vi "ENPH354_LabTracers2.vi"() -> ()   [LabVIEW 2020]
uses:
  1e4b00a4-0517-4322-bb3b-720fe8f45536.vi
  <vilib>/MakerHub/LINX/Public/Peripherals/PWM/PWM Set Duty Cycle 1 Chan.vi
  <vilib>/MakerHub/LINX/Public/Peripherals/Digital/Digital Write 1 Chan.vi
  75366657-9a63-4780-a10d-0fe28d3ec2d1.vi
  8bd6eaf3-79a2-4ca0-8ca0-17b2d510817e.vi
  <vilib>/MakerHub/LINX/Public/Peripherals/Analog/Analog Read 1 Chan.vi
  ab133cba-5ad7-442c-8e32-8a5f556f998e.vi
  <vilib>/MakerHub/LINX/Public/Peripherals/Digital/Digital Write N Chans.vi
  <vilib>/MakerHub/LINX/Public/Peripherals/Analog/Analog Read N Chans.vi
  <vilib>/MakerHub/LINX/Private/Local IO/LinxDigitalWrite.vi
  <vilib>/MakerHub/LINX/Public/Utilities/Check Channel.vi
  <vilib>/MakerHub/LINX/Private/Local IO/LinxAnalogRead.vi
  <vilib>/MakerHub/LINX/Public/Utilities/Open Serial.vi
  <vilib>/MakerHub/LINX/Public/Peripherals/PWM/PWM Set Duty Cycle N Chans.vi
  <vilib>/MakerHub/LINX/Private/Utilties/Generate Error.vi
  <vilib>/MakerHub/LINX/LMH-LINX.lvlib
panel:
  in  "Final Motor Angle [deg]":dbl
  in  "Initial Motor Angle [deg]":dbl
  in  "Motor Step Size [deg]":dbl
  in  "Voltage Step Size [V]":dbl
  out "PCE(n) [%]":dbl
  out "R_sh [Ohm]":dbl
  out "R_s [Ohm]":dbl
  out "FF":dbl
  out "V_oc [V]":dbl
  out "I_sc [A]":dbl
  out "Index":dbl
  out "Light Index":dbl
  out "Dark Index":dbl
  out "AVG Current SC [mA]":dbl
  out "AVG Current Light [mA]":dbl
  out "AVG Current Dark [mA]":dbl
  out "Duty Cycle":dbl
  out "AVG Bias V":dbl
  in  "Save Incident Angle Data":path
  in  "Save Dark IV Data":path
  in  "Save Light IV SCPE":path
  in  "Save Light IV Data":path
  in  "Skip Light":bool
  in  "Skip L&D":bool
  in  "Skip Dark":bool
  out "Short Circuit Current vs Incident Angle":cluster{"X":dbl[], "Y":dbl[]}[](graph)
  in  "stop 2":bool
  out "LED On":bool
  out "Light IV":cluster{"X":dbl[], "Y":dbl[]}[](graph)
  out "error out":errorcluster
  in  "stop":bool
  out "Bias Voltage":dbl(graph)
  out "Dark IV":cluster{"X":dbl[], "Y":dbl[]}[](graph)
  # "Press the \"Skip\" before executing"
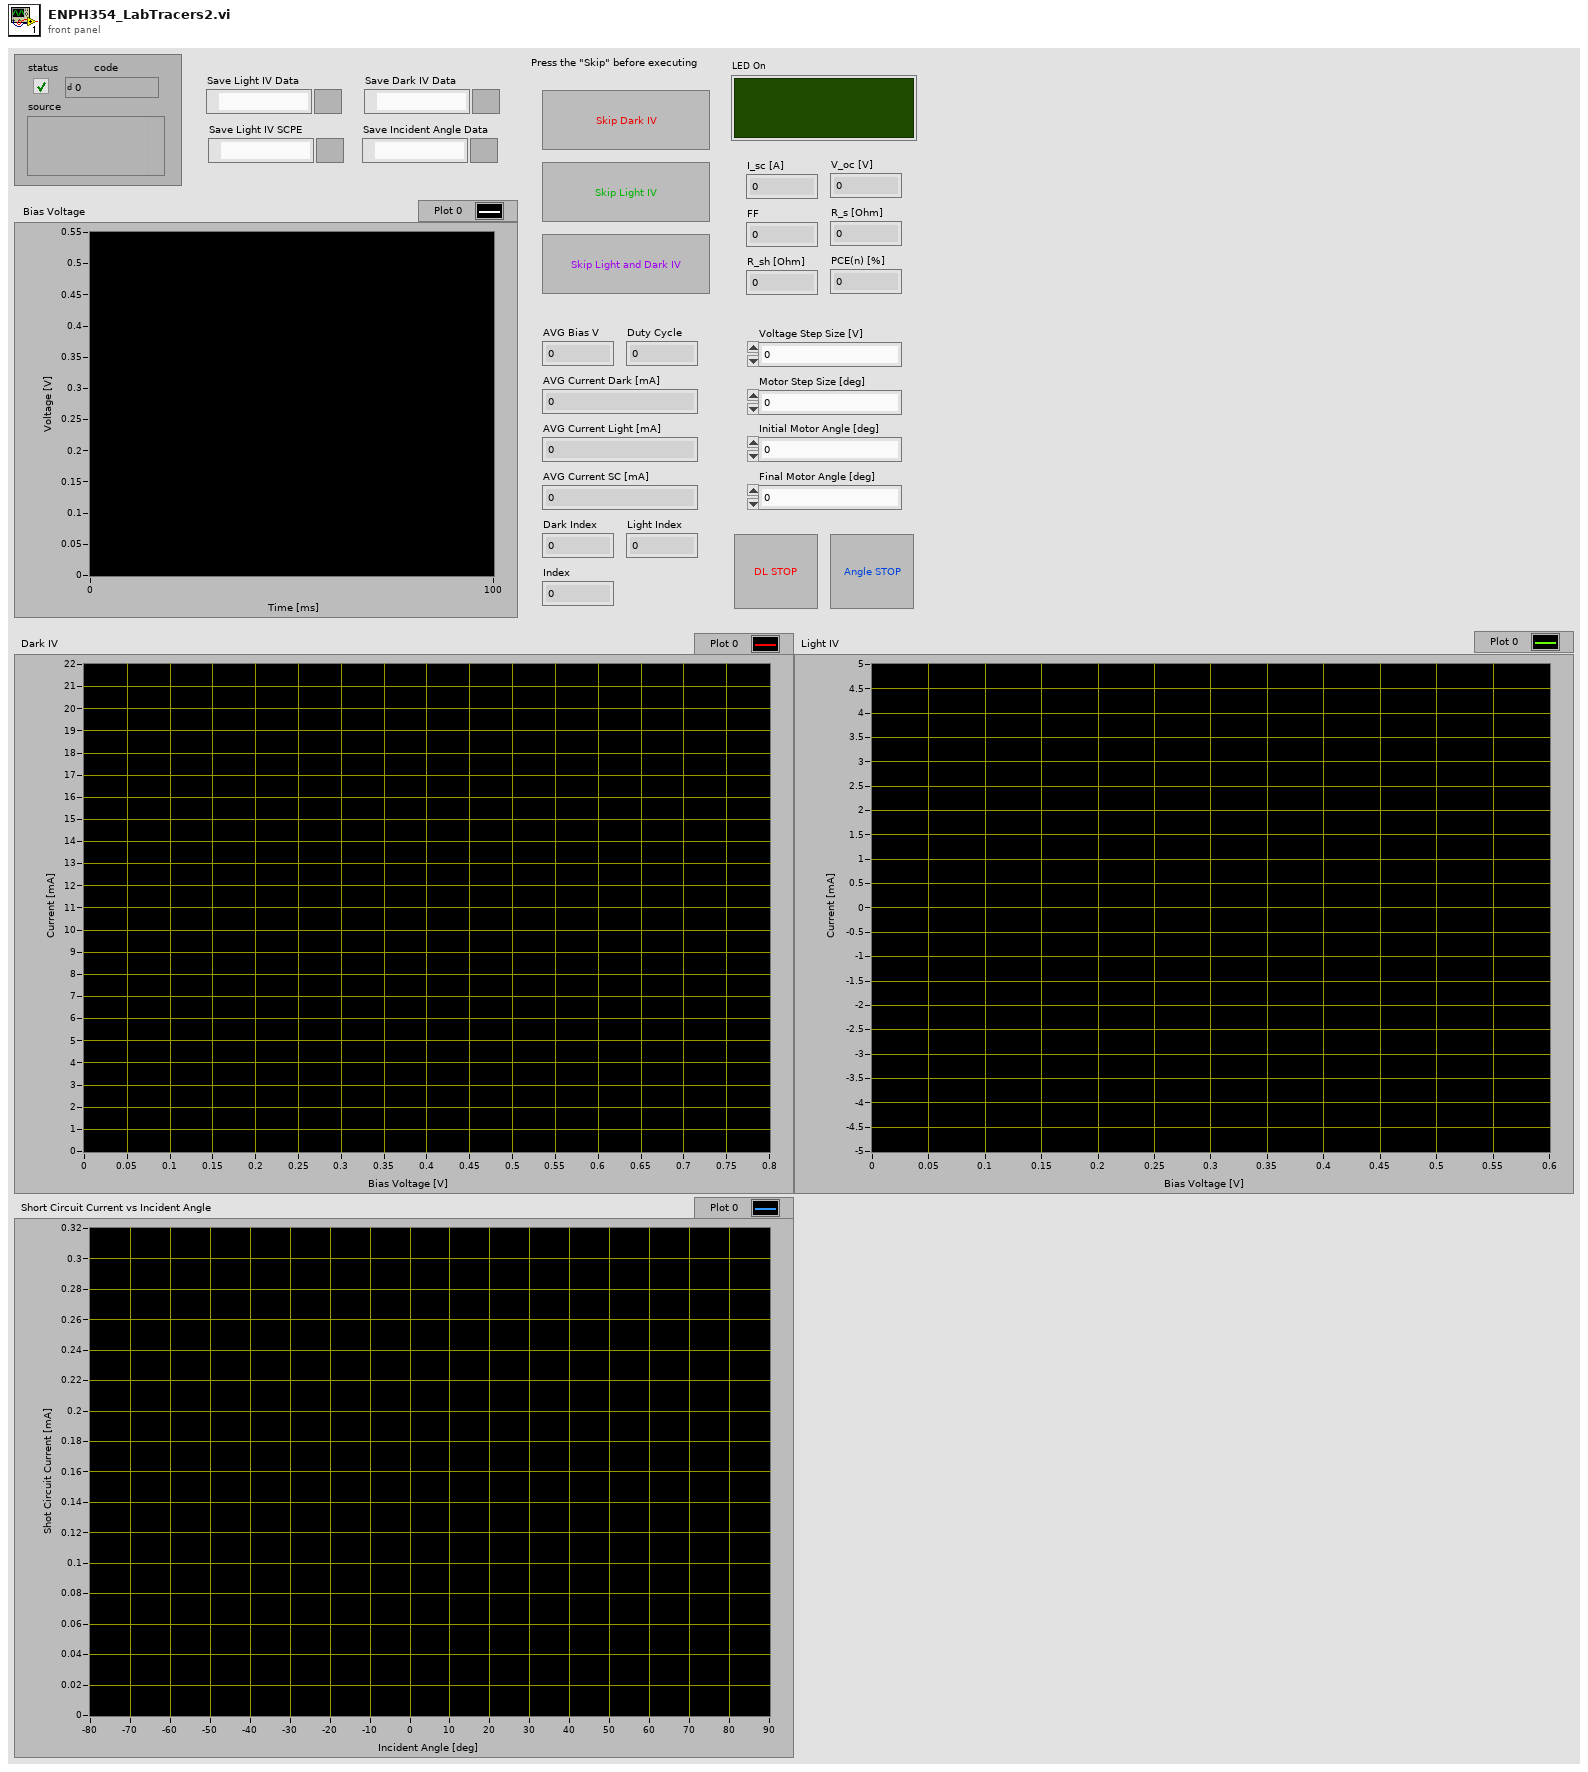
[diagram p1: front panel]
types:
  T1 = typedef "LMH-LINX.lvlib/LINX Ref.ctl" = cluster{"IO":T2, "Interface":T3, "LINX Device Config":T4}
  T2 = typedef "LMH-LINX.lvlib/Platform.ctl" = enum16{"Remote", "Local"}
  T3 = typedef "LMH-LINX.lvlib/Interface.ctl" = enum16{"Serial", "TCP"}
  T4 = typedef "LMH-LINX.lvlib/Device.lvlib/LINX Device Config.ctl" = cluster{"Interface":T3, "COM Port":refnum<visa-resource-name>, "TCP Configuration":T5, "Device Family":u8, "Device ID":u8, "Device Name":string, "TCP Ref":refnum<k5>, "Channels":T6}
  T5 = typedef "LMH-LINX.lvlib/Device.lvlib/TCP Config.ctl" = cluster{"IP Address":string, "Port":u16}
  T6 = typedef "LMH-LINX.lvlib/Channels.ctl" = cluster{"DI":u8[], "DO":u8[], "AI":u8[], "AO":u8[], "PWM":u8[], "QE":u8[], "UART":u8[], "I2C 2":u8[], "SPI":u8[], "CAN":u8[], "Servo":u8[], "AI Ref (V)":dbl, "AI Resolution (Bits)":u8, "AO Ref (V)":dbl, "AO Resolution (Bits)":u8}
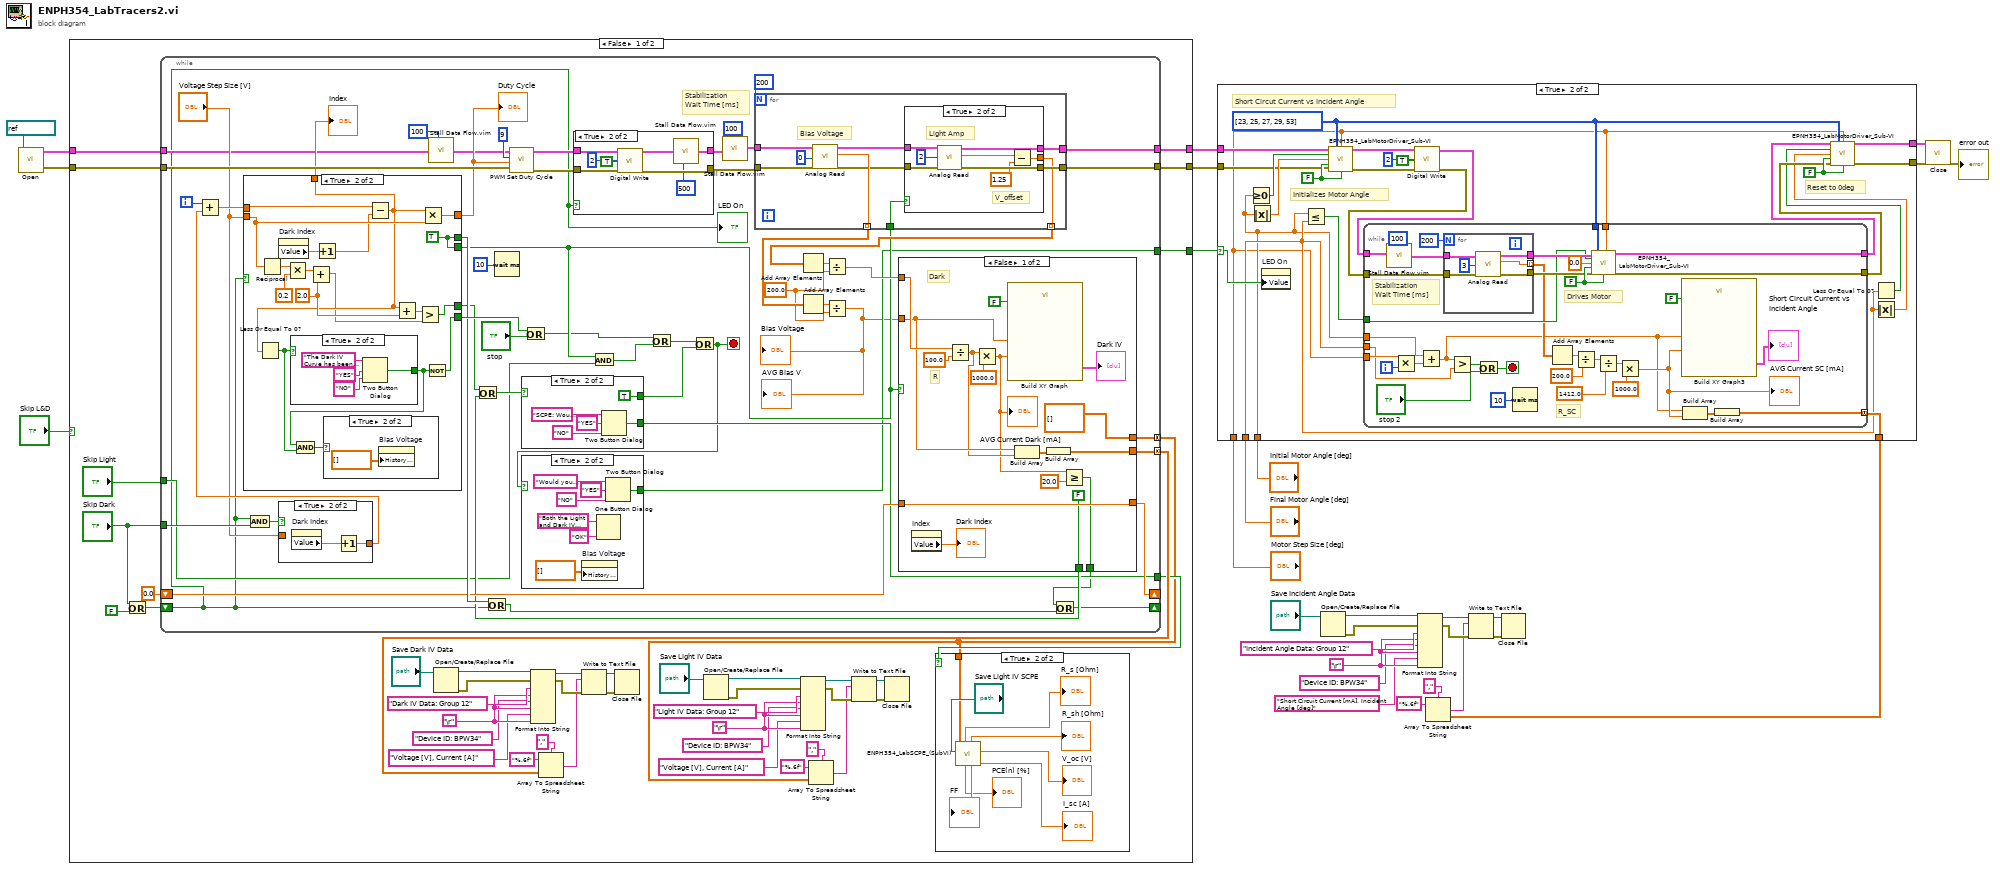
[diagram p0: block diagram]
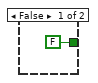
[diagram p3: hidden frame]
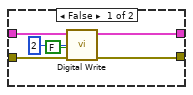
[diagram p4: hidden frame]
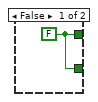
[diagram p5: hidden frame]
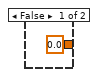
[diagram p6: hidden frame]
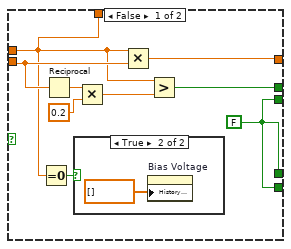
[diagram p7: hidden frame]
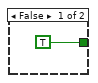
[diagram p10: hidden frame]
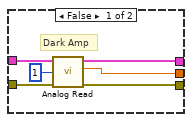
[diagram p11: hidden frame]
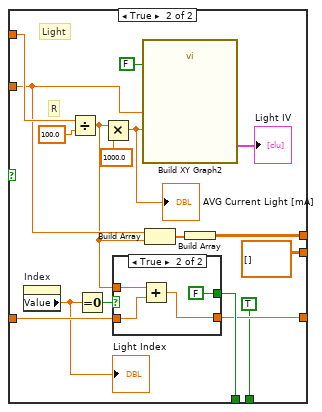
[diagram p12: hidden frame]
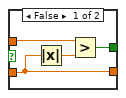
[diagram p13: hidden frame]
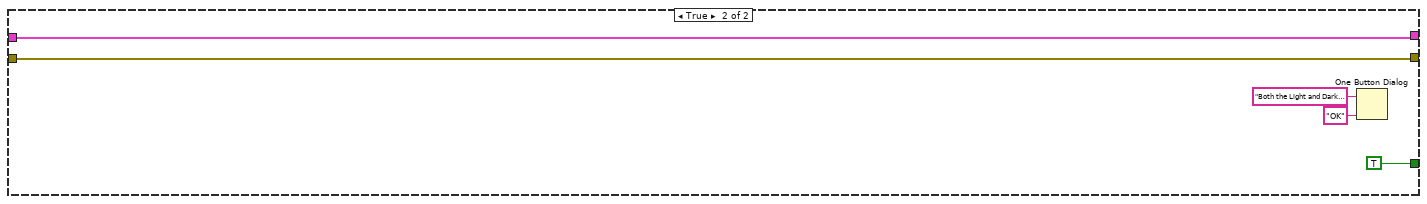
[diagram p14: hidden frame]
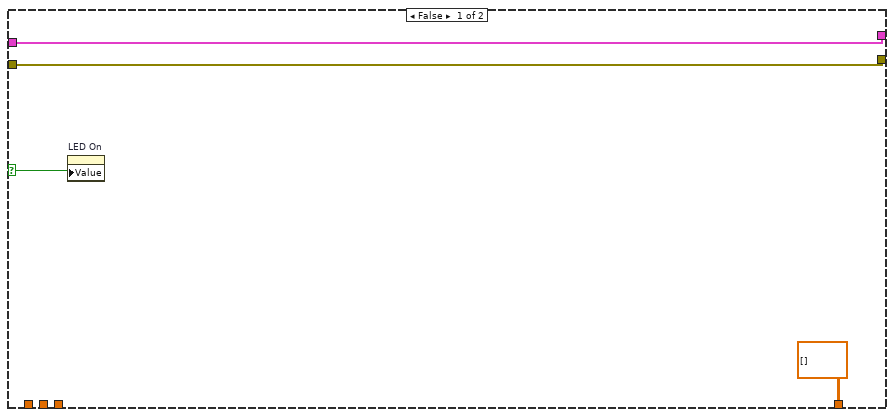
[diagram p15: hidden frame]
diagram:
  w10 = "\r"
  n1 = call-poly <vilib>:"Open.vi"("Serial Port"=refnum<visa-resource-name> "COM4") -> ("Error Out"=w26:errorcluster, "LINX Resource"=w27:T1)  [unwired: 8 in, 1 out]
  n2 = case shown="False" "Skip L&D" {
    tunnel: w27 -> [w69 w265]
    tunnel: w26 -> [w68 w264]
    tunnel: [w37 w265] -> w24
    tunnel: [w36 w264] -> w23
    tunnel: [w35 TRUE ("T button?")] -> w22
    frame False {
      w42 = "\r"
      w55 = "\r"
      n3 = Or(x="Skip Dark", y=FALSE) -> (x .or. y?=w67:bool)
      n4 = while {
        tunnel: w69 -> [w80]
        tunnel: w68 -> [w128]
        tunnel: [w124] -> w37
        tunnel: [w127] -> w36
        shift-right: [w99] -> _
        shift-left: w67 -> [w79]
        tunnel: "Skip Dark" -> [w109]
        tunnel: [w108] -> w29 mode=concatenating
        shift-right: [w107] -> _
        shift-left: 0.0 -> [w106]
        tunnel: [w101] -> w38
        tunnel: [w100] -> w39 mode=concatenating
        tunnel: [w89] -> w35
        tunnel: "Skip Light" -> [w91]
        i -> [w112]
        stop <- w88 stop-if-true
        w118 = 200.0 ("y")
        # "Stabilization\nWait Time [ms]"
        n5 = And(x=w79, y=w109) -> (x .and. y?=w110:bool)
        n6 = case shown="True" w110 {
          tunnel: "Voltage Step Size [V]" -> [_ _]
          tunnel: [0.0 w161] -> w111
          frame False {
          }
          frame True {
            n7 = property on="Dark Index" class="DigNum (strict)"() -> ("Value"=w160:dbl)  [unwired: 2 in, 2 out]
            n8 = Increment(x=w160) -> (x+1=w161:dbl)
          }
        }
        n9 = Add(x=w112, y=w111) -> (x+y=w113:dbl)
        n10 = case shown="True" w79 {
          tunnel: [w168 w188] -> w114
          tunnel: w113 -> [w163 w179]
          tunnel: "Voltage Step Size [V]" -> [w169 w178]
          tunnel: [w170 w189] -> w85
          tunnel: [w167 w188] -> w90
          tunnel: [w167 w187] -> w115
          tunnel: [w167 w186] -> w103
          tunnel: [w163 w175] -> w84
          frame False {
            w167 = FALSE
            n11 = Equal To 0?(x=w163) -> (x = 0?=w164:bool)
            n12 = Reciprocal(x=w169) -> (1/x=w166:dbl)
            n13 = case shown="True" w164 {
              frame False {
              }
              frame True {
                n14 = property on="Bias Voltage" class="WFChart (strict)"("History Data"=dbl[] []) -> ()  [unwired: 2 in, 2 out]
              }
            }
            n15 = Multiply(x=w166, y=0.2) -> (x*y=w162:dbl)
            n16 = Multiply(x=w163, y=w169) -> (x*y=w170:dbl)
            n17 = Greater?(x=w163, y=w162) -> (0:w168:bool)
          }
          frame True {
            w177 = 2.0 ("y")
            w188 = TRUE
            n18 = Reciprocal(x=w178) -> (1/x=w181:dbl)
            n19 = property on="Dark Index" class="DigNum (strict)"() -> ("Value"=w172:dbl)  [unwired: 2 in, 2 out]
            n20 = Multiply(x=w181, y=0.2) -> (x*y=w180:dbl)
            n21 = Add(x=w180, y=w177) -> (x+y=w174:dbl)
            n22 = Increment(x=w172) -> (x+1=w173:dbl)
            n23 = Subtract(x=w179, y=w173) -> (x-y=w175:dbl)
            n24 = Less Or Equal To 0?(x=w175) -> (x <= 0?=w176:bool)
            n25 = case shown="True" w176 {
              tunnel: [TRUE ("T button?") w193] -> w183
              frame False {
              }
              frame True {
                n26 = Two Button Dialog(message="The Dark IV Curve has been taken.\nWould you like to take the Light IV Curve?\n(NO: Terminates the program)", 1:"NO" ("F button name (\"Cancel\")"), 2:"YES" ("T button name (\"OK\")")) -> (T button?=w193:bool)
              }
            }
            n27 = And(x=w183, y=w176) -> (x .and. y?=w184:bool)
            n28 = case shown="True" w184 {
              frame False {
              }
              frame True {
                n29 = property on="Bias Voltage" class="WFChart (strict)"("History Data"=dbl[] []) -> ()  [unwired: 2 in, 2 out]
              }
            }
            n30 = Add(x=w175, y=w177) -> (x+y=w185:dbl)
            n31 = Greater?(x=w185, y=w174) -> (0:w186:bool)
            n32 = Multiply(x=w175, y=w178) -> (x*y=w189:dbl)
            n33 = Not(x=w183) -> (.not. x?=w187:bool)
          }
        }
        "Duty Cycle" <- w85
        "Index" <- w84
        n34 = call "Stall Data Flow.vim"("value in"=w80, "milliseconds to wait"=u32 100) -> ("value out"=w81:T1)  [unwired: 1 out]
        n35 = Or(x=w114, y=w79) -> (x .or. y?=w87:bool)
        n36 = Wait (ms)(milliseconds to wait=u32 10) -> ()  [unwired: 1 out]
        n37 = call-poly <vilib>:"PWM Set Duty Cycle.vi"("Error In"=w128, "Duty Cycle (0-1)"=w85, "PWM Channel"=u8 9, "LINX Resource"=w81) -> ("Error Out"=w96:errorcluster, "LINX Resource"=w97:T1)  [unwired: 6 in]
        n38 = Or(x=w115, y="stop") -> (x .or. y?=w78:bool)
        n39 = case shown="True" w79 {
          tunnel: w97 -> [w140 w149]
          tunnel: w96 -> [w139 w148]
          tunnel: [w142 w146] -> w95
          tunnel: [w141 w150] -> w94
          frame False {
            n40 = call-poly <vilib>:"Digital Write.vi"("Error In"=w139, "Output Value"=FALSE, "DO Channel"=u8 2, "LINX Resource"=w140) -> ("Error Out"=w141:errorcluster, "LINX Resource"=w142:T1)  [unwired: 6 in]
          }
          frame True {
            n41 = call-poly <vilib>:"Digital Write.vi"("Error In"=w148, "Output Value"=TRUE, "DO Channel"=u8 2, "LINX Resource"=w149) -> ("Error Out"=w150:errorcluster, "LINX Resource"=w147:T1)  [unwired: 6 in]
            n42 = call "Stall Data Flow.vim"("value in"=w147, "milliseconds to wait"=u32 500) -> ("value out"=w146:T1)  [unwired: 1 out]
          }
        }
        n43 = And(x=w90, y=w91) -> (x .and. y?=w92:bool)
        n44 = Or(x=w78, y=w92) -> (x .or. y?=w93:bool)
        n45 = call "Stall Data Flow.vim"("value in"=w95, "milliseconds to wait"=u32 100) -> ("value out"=w125:T1)  [unwired: 1 out]
        n46 = for {
          N: 200 -> [_]
          tunnel: [w202] -> w124
          tunnel: [w201] -> w127
          tunnel: w94 -> [w197]
          tunnel: w125 -> [w198]
          tunnel: [w205] -> w120 mode=indexing
          tunnel: [w200] -> w122 mode=indexing
          tunnel: w90 -> [w196]
          # "Bias Voltage"
          n47 = call-poly <vilib>:"Analog Read.vi"("Error In"=w197, "Analog Channel"=u8 0, "LINX Resource"=w198) -> ("Error Out"=w203:errorcluster, "Voltage"=w205:dbl, "LINX Resource"=w204:T1)  [unwired: 5 in, 1 out]
          n48 = case shown="True" w196 {
            tunnel: w204 -> [w208 w218]
            tunnel: [w210 w217] -> w202
            tunnel: w203 -> [w207 w216]
            tunnel: [w209 w215] -> w201
            tunnel: [w206 w213] -> w200
            frame False {
              # "Dark Amp"
              n49 = call-poly <vilib>:"Analog Read.vi"("Error In"=w207, "Analog Channel"=u8 1, "LINX Resource"=w208) -> ("Error Out"=w209:errorcluster, "Voltage"=w206:dbl, "LINX Resource"=w210:T1)  [unwired: 5 in, 1 out]
            }
            frame True {
              # "V_offset"
              # "Light Amp"
              n50 = call-poly <vilib>:"Analog Read.vi"("Error In"=w216, "Analog Channel"=u8 2, "LINX Resource"=w218) -> ("Error Out"=w215:errorcluster, "Voltage"=w214:dbl, "LINX Resource"=w217:T1)  [unwired: 5 in, 1 out]
              n51 = Subtract(x=w214, y=1.25) -> (x-y=w213:dbl)
            }
          }
        }
        n52 = Add Array Elements(numeric array=w122) -> (sum=w123:dbl)
        n53 = Add Array Elements(numeric array=w120) -> (sum=w121:dbl)
        n54 = Divide(x=w123, y=w118) -> (x/y=w119:dbl)
        n55 = Divide(x=w121, y=w118) -> (x/y=w86:dbl)
        "Bias Voltage" <- w86
        "AVG Bias V" <- w86
        n56 = case shown="False" w90 {
          tunnel: w119 -> [w231 w249]
          tunnel: w86 -> [w227 w247]
          tunnel: [dbl[][] [] w245] -> w108
          tunnel: [FALSE w243] -> w102
          tunnel: w106 -> [w229 w242]
          tunnel: [w229 w241] -> w107
          tunnel: [w225 dbl[][] []] -> w100
          tunnel: [w222 TRUE] -> w98
          frame False {
            # "Dark"
            # "R"
            n57 = property on="Index" class="DigNum (strict)"() -> ("Value"=→"Dark Index":dbl)  [unwired: 2 in, 2 out]
            n58 = Divide(x=w231, y=100.0) -> (x/y=w226:dbl)
            n59 = Multiply(x=w226, y=1000.0) -> (x*y=w221:dbl)
            "AVG Current Dark [mA]" <- w221
            n60 = call "Build XY Graph"("Reset"=FALSE, "Y Input"=w221, "X Input"=w227) -> ("XY Graph"=→"Dark IV":cluster{"X":dbl[], "Y":dbl[]}[])  [unwired: 7 in, 1 out]
            n61 = Build Array(w227, w226) -> (w228:dbl[])
            n62 = Build Array(w228) -> (w225:dbl[][])
            n63 = Greater Or Equal?(x=w221, y=20.0) -> (x >= y?=w222:bool)
          }
          frame True {
            # "R"
            # "Light"
            n64 = property on="Index" class="DigNum (strict)"() -> ("Value"=w236:dbl)  [unwired: 2 in, 2 out]
            "Light Index" <- w236
            n65 = Divide(x=w249, y=100.0) -> (x/y=w244:dbl)
            n66 = Equal To 0?(x=w236) -> (x = 0?=w240:bool)
            n67 = Multiply(x=w244, y=1000.0) -> (x*y=w237:dbl)
            "AVG Current Light [mA]" <- w237
            n68 = case shown="True" w240 {
              tunnel: w244 -> [w255 w258]
              tunnel: [w253 FALSE] -> w243
              tunnel: w242 -> [w254 w260]
              tunnel: [w254 w259] -> w241
              frame False {
                n69 = Absolute Value(x=w254) -> (abs(x)=w256:dbl)
                n70 = Greater?(x=w255, y=w256) -> (0:w253:bool)
              }
              frame True {
                n71 = Add(x=w258, y=w260) -> (x+y=w259:dbl)
              }
            }
            n72 = call "Build XY Graph2"("Reset"=FALSE, "Y Input"=w237, "X Input"=w247) -> ("XY Graph"=→"Light IV":cluster{"X":dbl[], "Y":dbl[]}[])  [unwired: 7 in, 1 out]
            n73 = Build Array(w247, w244) -> (w246:dbl[])
            n74 = Build Array(w246) -> (w245:dbl[][])
          }
        }
        n75 = Or(x=w103, y=w102) -> (x .or. y?=w104:bool)
        n76 = case shown="True" w104 {
          tunnel: [w153 TRUE ("true")] -> w105
          tunnel: [w153 w155] -> w101
          frame False {
            w153 = FALSE ("true")
          }
          frame True {
            n77 = Two Button Dialog(message="SCPE: Would you like to calculate the 6 solar cell parameters for the light IV curve?", 1:"NO" ("F button name (\"Cancel\")"), 2:"YES" ("T button name (\"OK\")")) -> (T button?=w155:bool)
          }
        }
        n78 = Or(x=w93, y=w105) -> (x .or. y?=w88:bool)
        n79 = case shown="True" w88 {
          tunnel: [FALSE ("T button?") w135] -> w89
          frame False {
          }
          frame True {
            n80 = property on="Bias Voltage" class="WFChart (strict)"("History Data"=dbl[] []) -> ()  [unwired: 2 in, 2 out]
            n81 = One Button Dialog(message="Both the Light and Dark IV Curves have been taken.", button name ("OK")="OK") -> ()  [unwired: 1 out]
            n82 = Two Button Dialog(message="Would you like to calculate the Short Circuit Current vs Incident Angle?", 1:"NO" ("F button name (\"Cancel\")"), 2:"YES" ("T button name (\"OK\")")) -> (T button?=w135:bool)
          }
        }
        n83 = Or(x=w98, y=w87) -> (x .or. y?=w99:bool)
        "LED On" <- w79
      }
      n84 = Open/Create/Replace File(file path (use dialog)="Save Dark IV Data") -> (refnum out=w52:refnum<file>, error out=w49:errorcluster)  [unwired: 5 in, 1 out]
      n85 = Format Into String(initial string=w52, error in=w49, "Dark IV Data: Group 12" ("input 1"), w42, "Device ID: BPW34" ("input 3"), w42, "Voltage [V], Current [A]", w42) -> (resulting string=w51:refnum<file>, error out=w48:errorcluster)  [unwired: 1 in]
      n86 = Array To Spreadsheet String(delimiter (Tab)=",", array=w39, 3:"%.6f" ("format string")) -> (spreadsheet string=w46:string)
      n87 = Write to Text File(file (use dialog)=w51, text=w46, error in=w48) -> (refnum out=w50:refnum<file>, error out=w47:errorcluster)  [unwired: 1 in, 1 out]
      n88 = Close File(refnum=w50, error in=w47) -> ()  [unwired: 2 out]
      n89 = Open/Create/Replace File(file path (use dialog)="Save Light IV Data") -> (refnum out=w65:refnum<file>, error out=w62:errorcluster)  [unwired: 5 in, 1 out]
      n90 = Format Into String(initial string=w65, error in=w62, "Light IV Data: Group 12" ("input 1"), w55, "Device ID: BPW34" ("input 3"), w55, "Voltage [V], Current [A]", w55) -> (resulting string=w64:refnum<file>, error out=w61:errorcluster)  [unwired: 1 in]
      n91 = Array To Spreadsheet String(delimiter (Tab)=",", array=w29, 3:"%.6f" ("format string")) -> (spreadsheet string=w59:string)
      n92 = Write to Text File(file (use dialog)=w64, text=w59, error in=w61) -> (refnum out=w63:refnum<file>, error out=w60:errorcluster)  [unwired: 1 in, 1 out]
      n93 = Close File(refnum=w63, error in=w60) -> ()  [unwired: 2 out]
      n94 = case shown="True" w38 {
        tunnel: w29 -> [_ w70]
        frame False {
        }
        frame True {
          n95 = call "ENPH354_LabSCPE_(SubVI).vi"("Save Data"="Save Light IV SCPE", "Array"=w70) -> ("I_sc [A]"=→"I_sc [A]":dbl, "V_oc [V]"=→"V_oc [V]":dbl, "FF"=→"FF":dbl, "R_sh [Ohm]"=→"R_sh [Ohm]":dbl, "PCE(n)"=→"PCE(n) [%]":dbl, "R_s [Ohm]"=→"R_s [Ohm]":dbl)  [unwired: 2 in, 2 out]
        }
      }
    }
    frame True {
      n96 = One Button Dialog(message="Both the Light and Dark IV Curves have been skipped.", button name ("OK")="OK") -> ()  [unwired: 1 out]
    }
  }
  n97 = case shown="True" w22 {
    selector: w22 -> [w266 w285]
    tunnel: "Motor Step Size [deg]" -> [_ w274]
    tunnel: w24 -> [w269 w290]
    tunnel: "Final Motor Angle [deg]" -> [_ w280]
    tunnel: "Initial Motor Angle [deg]" -> [_ w279]
    tunnel: w23 -> [w268 w289]
    tunnel: [w269 w288] -> w21
    tunnel: [w268 w287] -> w1
    tunnel: [dbl[][] [] w286] -> w3
    frame False {
      n98 = property on="LED On" class="Bool (strict)"("Value"=w266) -> ()  [unwired: 2 in, 2 out]
    }
    frame True {
      w291 = FALSE ("Run Continuous in")
      w275 = i32[] [23, 25, 27, 29, 53] ("Array")
      w294 = FALSE ("Run Continuous in")
      # "Short Circut Current vs Incident Angle"
      # "Reset to 0deg"
      # "Initializes Motor Angle"
      n99 = Greater Or Equal To 0?(x=w279) -> (x >= 0?=w293:bool)
      n100 = Absolute Value(x=w279) -> (abs(x)=w292:dbl)
      n101 = property on="LED On" class="Bool (strict)"("Value"=w285) -> ()  [unwired: 2 in, 2 out]
      n102 = Less Or Equal?(x=w279, y=w280) -> (x <= y?=w278:bool)
      n103 = call "EPNH354_LabMotorDriver_Sub-VI.vi"("LINX Resource in"=w290, "Array"=w275, "Step Size in"=w274, "Run Clockwise in"=w293, "Rotation Range in"=w292, "Run Continuous in"=w294, "error in (no error)"=w289, "stop in"=w294) -> ("LINX Resource out"=w282:T1, "error out"=w281:errorcluster)  [unwired: 6 in]
      n104 = call-poly <vilib>:"Digital Write.vi"("Error In"=w281, "Output Value"=TRUE, "DO Channel"=u8 2, "LINX Resource"=w282) -> ("Error Out"=w277:errorcluster, "LINX Resource"=w276:T1)  [unwired: 6 in]
      n105 = while {
        tunnel: w276 -> [w329]
        tunnel: w277 -> [w327]
        tunnel: w278 -> [w321]
        tunnel: w279 -> [w317]
        tunnel: w280 -> [w295]
        tunnel: w274 -> [w319]
        tunnel: [w307] -> w273
        tunnel: [w306] -> w272
        tunnel: w274 -> [w305]
        tunnel: w275 -> [w304]
        tunnel: [w302] -> w286 mode=concatenating
        i -> [w316]
        stop <- w297 stop-if-true
        w325 = FALSE ("Run Continuous in")
        # "R_SC"
        # "Drives Motor"
        # "Stabilization\nWait Time [ms]"
        n106 = call "Stall Data Flow.vim"("value in"=w329, "milliseconds to wait"=u32 100) -> ("value out"=w328:T1)  [unwired: 1 out]
        n107 = Multiply(x=w319, y=w316) -> (x*y=w318:dbl)
        n108 = Add(x=w317, y=w318) -> (x+y=w296:dbl)
        n109 = for {
          N: 200 -> [_]
          tunnel: w328 -> [w331]
          tunnel: w327 -> [w335]
          tunnel: [w334] -> w323
          tunnel: [w333] -> w322
          tunnel: [w332] -> w312 mode=indexing
          n110 = call-poly <vilib>:"Analog Read.vi"("Error In"=w335, "Analog Channel"=u8 3, "LINX Resource"=w331) -> ("Error Out"=w333:errorcluster, "Voltage"=w332:dbl, "LINX Resource"=w334:T1)  [unwired: 5 in, 1 out]
        }
        n111 = Greater?(x=w296, y=w295) -> (0:w320:bool)
        n112 = Or(x=w320, y="stop 2") -> (x .or. y?=w297:bool)
        n113 = Wait (ms)(milliseconds to wait=u32 10) -> ()  [unwired: 1 out]
        n114 = Add Array Elements(numeric array=w312) -> (sum=w314:dbl)
        n115 = Divide(x=w314, y=200.0) -> (x/y=w311:dbl)
        n116 = call "EPNH354_LabMotorDriver_Sub-VI.vi"("LINX Resource in"=w323, "Array"=w304, "Step Size in"=w305, "Run Clockwise in"=w321, "Rotation Range in"=0.0, "Run Continuous in"=w325, "error in (no error)"=w322, "stop in"=w325) -> ("LINX Resource out"=w307:T1, "error out"=w306:errorcluster)  [unwired: 6 in]
        n117 = Divide(x=w311, y=1412.0) -> (x/y=w301:dbl)
        n118 = Multiply(x=w301, y=1000.0) -> (x*y=w299:dbl)
        "AVG Current SC [mA]" <- w299
        n119 = call "Build XY Graph3"("Reset"=FALSE, "Y Input"=w299, "X Input"=w296) -> ("XY Graph"=→"Short Circuit Current vs Incident Angle":cluster{"X":dbl[], "Y":dbl[]}[])  [unwired: 7 in, 1 out]
        n120 = Build Array(w296, w299) -> (w303:dbl[])
        n121 = Build Array(w303) -> (w302:dbl[][])
      }
      n122 = Less Or Equal To 0?(x=w280) -> (x <= 0?=w271:bool)
      n123 = Absolute Value(x=w280) -> (abs(x)=w270:dbl)
      n124 = call "EPNH354_LabMotorDriver_Sub-VI.vi"("LINX Resource in"=w273, "Array"=w275, "Step Size in"=w274, "Run Clockwise in"=w271, "Rotation Range in"=w270, "Run Continuous in"=w291, "error in (no error)"=w272, "stop in"=w291) -> ("LINX Resource out"=w288:T1, "error out"=w287:errorcluster)  [unwired: 6 in]
    }
  }
  n125 = Open/Create/Replace File(file path (use dialog)="Save Incident Angle Data") -> (refnum out=w20:refnum<file>, error out=w17:errorcluster)  [unwired: 5 in, 1 out]
  n126 = Format Into String(initial string=w20, error in=w17, "Incident Angle Data: Group 12" ("input 1"), w10, "Device ID: BPW34" ("input 3"), w10, "Short Circuit Current [mA], Incident Angle [deg]", w10) -> (resulting string=w19:refnum<file>, error out=w16:errorcluster)  [unwired: 1 in]
  n127 = Array To Spreadsheet String(delimiter (Tab)=",", array=w3, 3:"%.6f" ("format string")) -> (spreadsheet string=w14:string)
  n128 = Write to Text File(file (use dialog)=w19, text=w14, error in=w16) -> (refnum out=w18:refnum<file>, error out=w15:errorcluster)  [unwired: 1 in, 1 out]
  n129 = Close File(refnum=w18, error in=w15) -> ()  [unwired: 2 out]
  n130 = call <vilib>:"Close.vi"("Error In"=w1, "LINX Resource"=w21) -> ("Error Out"=→"error out":errorcluster)  [unwired: 9 in]
